vi "StringFormat.vi"(9 "UnitStr":string, 10 "MeasureValue":sgl format="%#.25f", 11 "TYPE":u8) -> (3 "WorkCurrent":string)   [LabVIEW 2016]
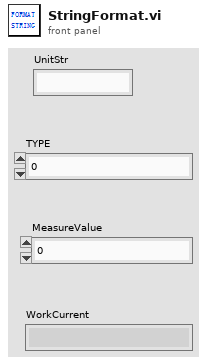
[diagram p1: front panel]
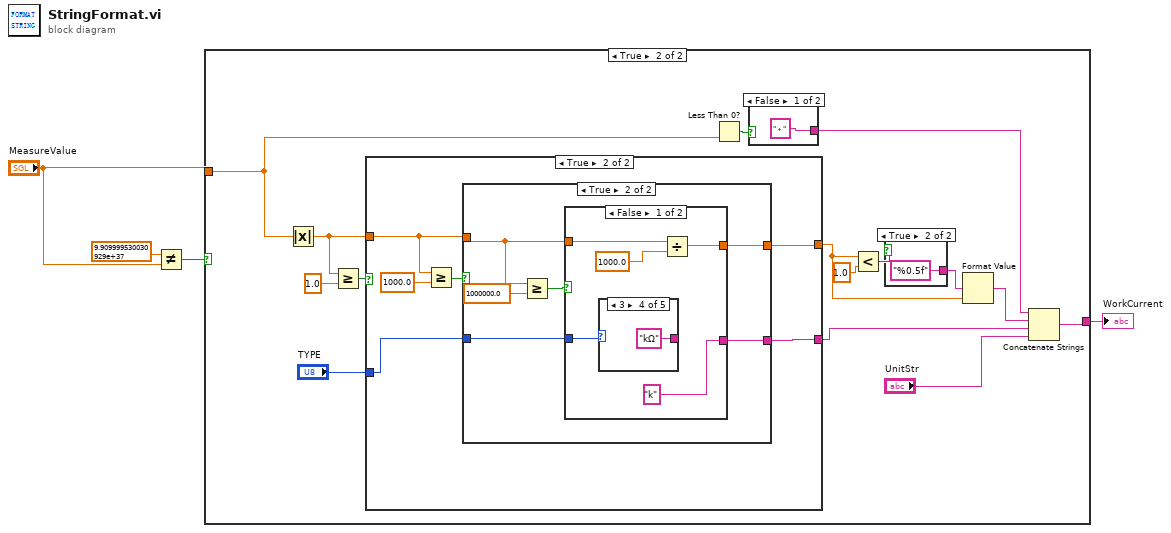
[diagram p0: block diagram]
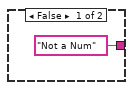
[diagram p2: hidden frame]
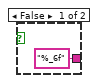
[diagram p3: hidden frame]
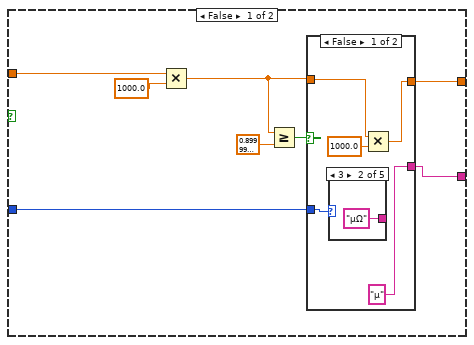
[diagram p4: hidden frame]
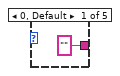
[diagram p5: hidden frame]
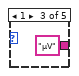
[diagram p6: hidden frame]
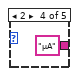
[diagram p7: hidden frame]
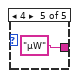
[diagram p8: hidden frame]
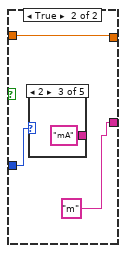
[diagram p9: hidden frame]
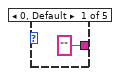
[diagram p10: hidden frame]
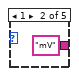
[diagram p11: hidden frame]
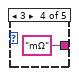
[diagram p12: hidden frame]
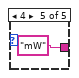
[diagram p13: hidden frame]
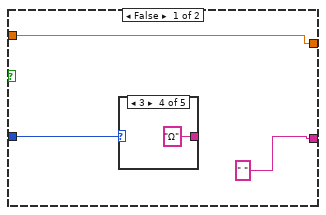
[diagram p14: hidden frame]
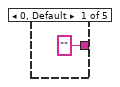
[diagram p15: hidden frame]
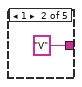
[diagram p16: hidden frame]
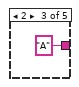
[diagram p17: hidden frame]
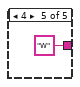
[diagram p18: hidden frame]
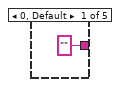
[diagram p19: hidden frame]
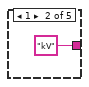
[diagram p20: hidden frame]
diagram:
  n1 = Not Equal?(x=sgl 9.91e+37 ("MeasureValue"), y="MeasureValue") -> (x != y?=w1:bool)
  n2 = case shown="True" w1 {
    tunnel: "MeasureValue" -> [_ w20]
    tunnel: ["Not a Num" w18] -> w4
    frame False {
    }
    frame True {
      n3 = Absolute Value(x=w20) -> (abs(x)=w11:sgl)
      n4 = Greater Or Equal?(x=w11, y=sgl 1.0) -> (x >= y?=w13:bool)
      n5 = case shown="True" w13 {
        tunnel: w11 -> [w28 w52]
        tunnel: [w30 w51] -> w9
        tunnel: [w29 w49] -> w19
        tunnel: "TYPE" -> [w27 w50]
        frame False {
          n6 = Multiply(x=w28, y=sgl 1000.0) -> (x*y=w24:sgl)
          n7 = Greater Or Equal?(x=w24, y=sgl 0.9) -> (x >= y?=w23:bool)
          n8 = case shown="False" w23 {
            tunnel: w24 -> [w33 w43]
            tunnel: [w34 w43] -> w30
            tunnel: ["μ" ("string") "m" ("string")] -> w29
            tunnel: w27 -> [w32 w42]
            frame False {
              n9 = case shown="3" w32 {
                tunnel: ["" ("string") "μΩ" ("string") "μV" ("string") "μA" ("string") "μW" ("string")] -> _
                frame 0, Default {
                }
                frame 3 {
                }
                frame 1 {
                }
                frame 2 {
                }
                frame 4 {
                }
              }
              n10 = Multiply(x=w33, y=sgl 1000.0) -> (x*y=w34:sgl)
            }
            frame True {
              n11 = case shown="2" w42 {
                tunnel: ["" ("string") "mV" ("string") "mA" ("string") "mΩ" ("string") "mW" ("string")] -> _
                frame 0, Default {
                }
                frame 1 {
                }
                frame 2 {
                }
                frame 3 {
                }
                frame 4 {
                }
              }
            }
          }
        }
        frame True {
          n12 = Greater Or Equal?(x=w52, y=sgl 1000.0) -> (x >= y?=w53:bool)
          n13 = case shown="True" w53 {
            tunnel: [w57 w68] -> w51
            tunnel: [" " ("string") w66] -> w49
            tunnel: w52 -> [w57 w64]
            tunnel: w50 -> [w56 w67]
            frame False {
              n14 = case shown="3" w56 {
                tunnel: ["" ("string") "V" ("string") "A" ("string") "Ω" ("string") "W" ("string")] -> _
                frame 0, Default {
                }
                frame 1 {
                }
                frame 2 {
                }
                frame 3 {
                }
                frame 4 {
                }
              }
            }
            frame True {
              n15 = Greater Or Equal?(x=w64, y=sgl 1000000.0) -> (x >= y?=w63:bool)
              n16 = case shown="False" w63 {
                tunnel: [w72 w81] -> w68
                tunnel: w67 -> [w71 w80]
                tunnel: ["k" ("string") "M" ("string")] -> w66
                tunnel: w64 -> [w70 w82]
                frame False {
                  n17 = case shown="3" w71 {
                    tunnel: ["" ("string") "kV" ("string") "kA" ("string") "kΩ" ("string") "kW" ("string")] -> _
                    frame 0, Default {
                    }
                    frame 1 {
                    }
                    frame 2 {
                    }
                    frame 3 {
                    }
                    frame 4 {
                    }
                  }
                  n18 = Divide(x=w70, y=sgl 1000.0) -> (x/y=w72:sgl)
                }
                frame True {
                  n19 = case shown="3" w80 {
                    tunnel: ["" ("string") "MΩ" ("string") "mW" ("string")] -> _
                    frame 0, Default {
                    }
                    frame 3 {
                    }
                    frame 4 {
                    }
                  }
                  n20 = Divide(x=w82, y=sgl 1000000.0) -> (x/y=w81:sgl)
                }
              }
            }
          }
        }
      }
      n21 = Less Than 0?(x=w20) -> (x < 0?=w17:bool)
      n22 = case shown="False" w17 {
        tunnel: ["＋" ("string") "－" ("string")] -> w16
        frame False {
        }
        frame True {
        }
      }
      n23 = Less?(x=w9, y=sgl 1.0) -> (x < y?=w7:bool)
      n24 = case shown="True" w7 {
        tunnel: ["%_6f" ("format string") "%0.5f" ("format string")] -> w14
        frame False {
        }
        frame True {
        }
      }
      n25 = Format Value(format string=w14, value (0)=w9) -> (output string=w15:string)  [unwired: 1 in]
      n26 = Concatenate Strings(w16, w15, w19, "UnitStr") -> (w18:string)
    }
  }
  "WorkCurrent" <- w4
